vi "MVE Write Setting.vi"(10 "value":string, 11 "key":string) -> (3 "Success":bool)   [LabVIEW 2016]
uses:
  <resource>/dialog/lvconfig.llb/LV Config Write String.vi
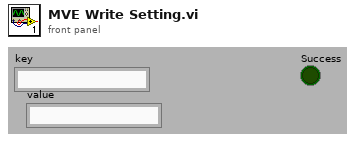
[diagram p1: front panel]
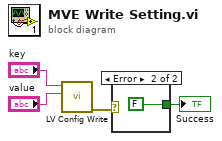
[diagram p0: block diagram]
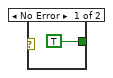
[diagram p2: hidden frame]
diagram:
  n1 = call-poly <resource>:"LV Config Write.vi"("value"="value", "key"="key") -> ("error out"=w2:errorcluster)  [unwired: 5 in]
  n2 = case shown="Error" w2 {
    tunnel: [TRUE FALSE] -> w1
    frame No Error {
    }
    frame Error {
    }
  }
  "Success" <- w1
